vi "drilling.vi"(8 "error in (no error)":errorcluster, 10 "relencoderdelay":i16, 11 "pulsewidth":i16) -> (0 "error out":errorcluster)   [LabVIEW 2015, in "SCANalone4x64.lvlib"]
doc: "__declspec(dllimport) void __stdcall drilling(short pulsewidth, short relencoderdelay);"
uses:
  <userlib>/SCANalone4x64/SCANalone4x64.lvlib
  <userlib>/SCANalone4x64/SCANalone4x64.dll
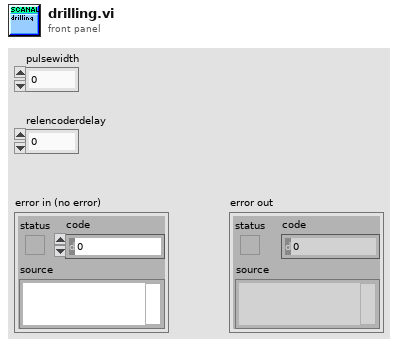
[diagram p1: front panel]
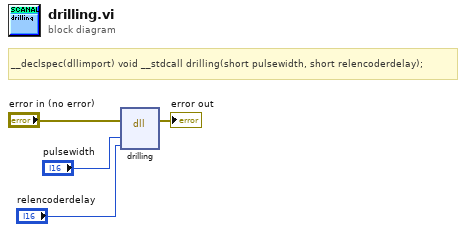
[diagram p0: block diagram]
diagram:
  # "__declspec(dllimport) void __stdcall drilling(short pulsewidth, short relencoderdelay);"
  n1 = dll-call lib="C:/Program Files/National Instruments/LabVIEW 2015/user.lib/SCANalone4x64/SCANalone4x64.*" fn="drilling"(error in="error in (no error)", "pulsewidth"="pulsewidth", "relencoderdelay"="relencoderdelay") -> (error out=→"error out":errorcluster)  [unwired: 5 in, 1 out]
